vi "Read gRPCid.vi"(8 "error in (no error)":errorcluster, 11 "iService in":refnum<class "iService.lvclass">) -> (0 "error out":errorcluster, 2 "gRPCid":T1, 3 "iService out":refnum<class "iService.lvclass">)   [LabVIEW 2019, in "gRPC-servicer.lvlib" / "iService.lvclass"]
uses:
  iService.lvclass
  <vilib>/gRPC/LabVIEW gRPC Library/Server API/typeDefs/grpcId.ctl
  iService.lvclass/iService.ctl
  <vilib>/gRPC/LabVIEW gRPC Library/gprc-lvsupport-release.lvlib
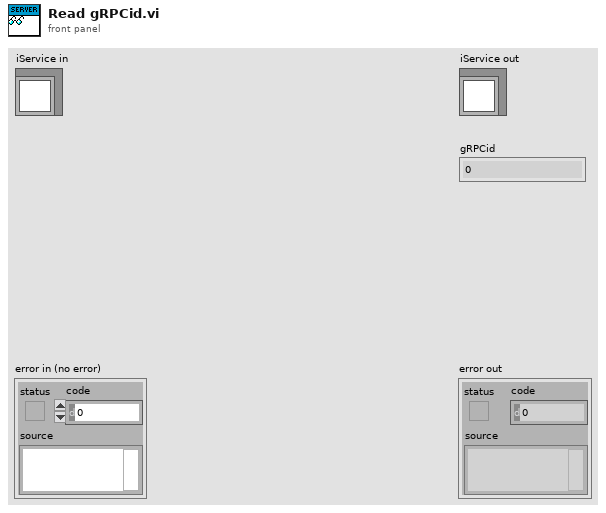
[diagram p1: front panel]
types:
  T1 = typedef "gprc-lvsupport-release.lvlib/grpcId.ctl" = u64
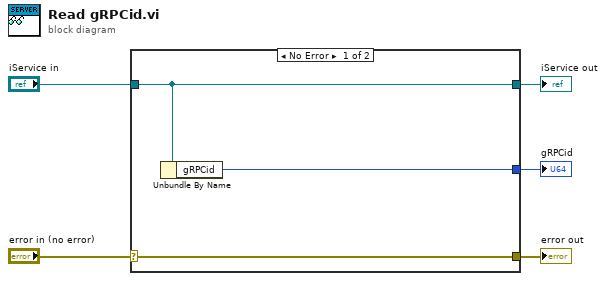
[diagram p0: block diagram]
diagram:
  n1 = case shown="No Error" "error in (no error)" {
    selector: "error in (no error)" -> [w8 w9]
    tunnel: [w8 w9] -> w4
    tunnel: [w7 w10] -> w2
    tunnel: "iService in" -> [w7 w10]
    tunnel: [w6 _] -> w1
    frame No Error {
      n2 = Unbundle By Name(w7) -> ("gRPCid"=w6:T1)
    }
    frame Error {
    }
  }
  "error out" <- w4
  "iService out" <- w2
  "gRPCid" <- w1
